vi "write_attributes.vi"(8 "error in (no error)":errorcluster, 10 "attributes":T1, 11 "KernelPCA in":refnum<class "KernelPCA.lvclass">) -> (0 "error out":errorcluster, 3 "KernelPCA out":refnum<class "KernelPCA.lvclass">)   [LabVIEW 2020, in "KernelPCA.lvclass"]
uses:
  KernelPCA.lvclass
  Controls/kernel_pca_attributes.ctl
  KernelPCA.lvclass/KernelPCA.ctl
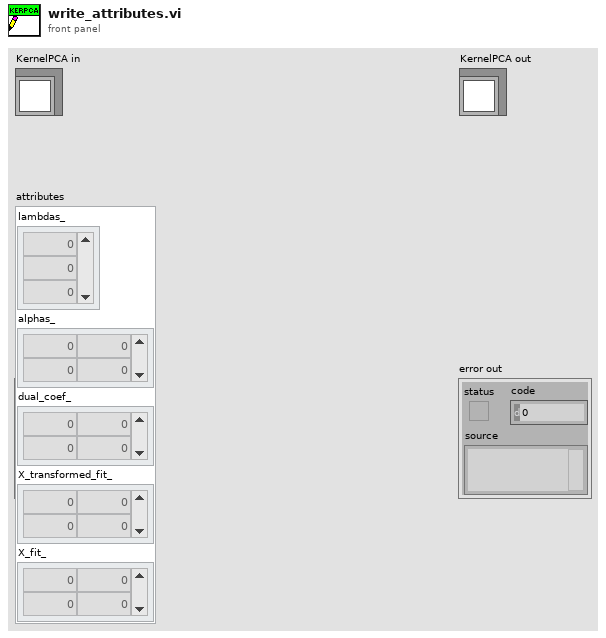
[diagram p1: front panel]
types:
  T1 = typedef "kernel_pca_attributes.ctl" = cluster{"lambdas_":dbl[], "alphas_":dbl[][], "dual_coef_":dbl[][], "X_transformed_fit_":dbl[][], "X_fit_":dbl[][]}
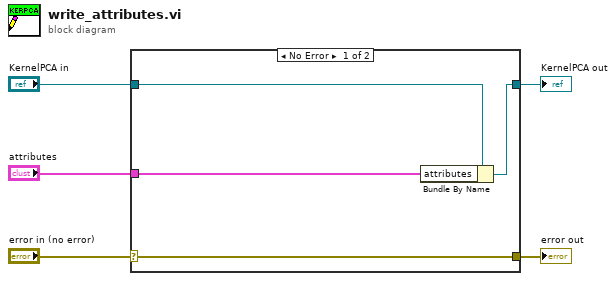
[diagram p0: block diagram]
diagram:
  n1 = case shown="No Error" "error in (no error)" {
    selector: "error in (no error)" -> [w9 w10]
    tunnel: [w9 w10] -> w4
    tunnel: [w7 w11] -> w2
    tunnel: "KernelPCA in" -> [w8 w11]
    tunnel: "attributes" -> [w6 _]
    frame No Error {
      n2 = Bundle By Name(cluster=w8, "attributes"=w6) -> (w7:refnum<class "KernelPCA.lvclass">)
    }
    frame Error {
    }
  }
  "error out" <- w4
  "KernelPCA out" <- w2
